vi "Draw Steering Frame Picture_Multiple Colors.vi"(5 "wheel colors":u32[](array[colorbox]), 6 "steering frame position":T1, 7 "drawing options":T2={"draw wheel states?"=FALSE, "highlight wheel index"=-1, "pixels per unit"=10.0, "draw forward velocity?"=FALSE, "velocity scale"=1.0}, 8 "error in (no error)":errorcluster, 9 "picture draw area size (pixels)":cluster{"width":u32, "height":u32}={"width"=500, "height"=500}, 10 "picture in":picture, 11 "steering frame in":refnum<class "NI_Robotics_Steering Frame.lvclass">) -> (0 "error out":errorcluster, 2 "picture out":picture, 3 "steering frame out":refnum<class "NI_Robotics_Steering Frame.lvclass">)   [LabVIEW 2017, in "NI_Robotics_Steering Picture.lvlib"]
doc: "Creates an image you can wire to a 2D picture control to visualize a steering frame on the front panel. The picture can display data about the directions and velocities at which wheels move."
uses:
  <vilib>/robotics/Utilities/Visualization/Steering Visualization/Steering Picture/NI_Robotics_Steering Picture.lvlib
  <vilib>/robotics/Steering/Steering Frame/NI_Robotics_Steering Frame.lvclass
  <vilib>/robotics/Utilities/Visualization/Steering Visualization/Steering Picture/Draw Steering Frame Options.ctl
  <vilib>/robotics/Utilities/Visualization/Steering Visualization/Steering Picture/Picture Info.ctl
  <vilib>/Utility/miscctls.llb/LVBoundsTypeDef.ctl
  <vilib>/robotics/Steering/Steering Frame/NI_Robotics_Steering Frame.lvclass/NI_Robotics_Steering Frame.ctl
  <vilib>/Analysis/coordinate.llb/2D Cartesian Coordinate Rotation (Array).vi
  <vilib>/Analysis/coordinate.llb/Angle Rotation with Same Angle (array).vi
  <vilib>/robotics/Utilities/Visualization/Steering Visualization/Steering Picture/Draw Arrow.vi
  <vilib>/robotics/Utilities/Visualization/Steering Visualization/Steering Picture/Draw Wheel Axle.vi
  <vilib>/robotics/Utilities/Visualization/Steering Visualization/Steering Picture/Draw Wheel Outline.vi
  <vilib>/robotics/Utilities/Visualization/Steering Visualization/Steering Picture/Draw Fixed Wheel Forward Velocity.vi
  <vilib>/robotics/Utilities/Visualization/Steering Visualization/Steering Picture/Draw Wedge.vi
  <vilib>/robotics/Utilities/Visualization/Steering Visualization/Steering Picture/Draw Steering Wheel Forward Velocity.vi
  <vilib>/Analysis/coordinate.llb/Angle Rotation (scalar).vi
  <vilib>/Analysis/coordinate.llb/2D Cartesian Coordinate Rotation (Scalar).vi
  <vilib>/robotics/Utilities/Visualization/Steering Visualization/Steering Picture/Global Position to Pixel.vi
  <vilib>/robotics/Utilities/Visualization/Steering Visualization/Steering Picture/Draw Caster Wheel Forward Velocity.vi
  <vilib>/robotics/Utilities/Visualization/Steering Visualization/Steering Picture/Draw Lines.vi
  <vilib>/Analysis/coordinate.llb/Wrap Angle (array).vi
  <vilib>/Analysis/coordinate.llb/Wrap Angle.vi
  <vilib>/Analysis/coordinate.llb/Wrap Angle (scalar).vi
  <vilib>/picture/picture.llb/Draw Line.vi
  <vilib>/picture/picture.llb/Move Pen.vi
  <vilib>/picture/picture.llb/Draw Point.vi
  <vilib>/picture/picture.llb/Draw Multiple Lines.vi
  <vilib>/robotics/Steering/Wheel/Get Wheel Information.vi
  <vilib>/robotics/Steering/Wheel/Get Omnidirectional Wheel Information.vi
  <vilib>/robotics/Steering/Wheel/Get Mecanum Wheel Information.vi
  <vilib>/robotics/Steering/Wheel/Get Caster Wheel Information.vi
  <vilib>/picture/pictutil.llb/Draw Circle by Radius.vi
  <vilib>/Utility/AngleManip/Radians to Degrees.vi
  <vilib>/Utility/AngleManip/Radians to Degrees (Scalar DBL).vi
  <vilib>/robotics/Steering/Wheel/Get Steering Wheel Information.vi
  <vilib>/robotics/Steering/Wheel/Get Fixed Wheel Information.vi
  <vilib>/robotics/Steering/Wheel/NI_Robotics_Wheel.lvclass
  <vilib>/Analysis/NI_AALPro.lvlib
  <vilib>/Analysis/NI_AAL_Angle.lvlib
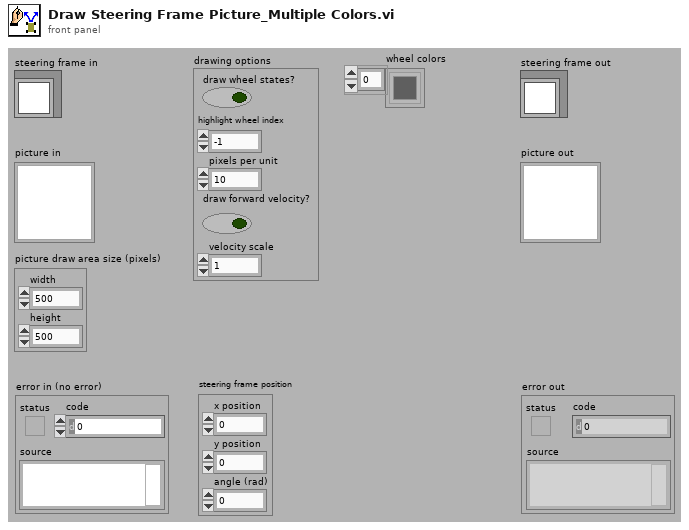
[diagram p1: front panel]
types:
  T1 = cluster{"x position":dbl, "y position":dbl, "angle (rad)":dbl}
  T2 = typedef "NI_Robotics_Steering Picture.lvlib/Draw Steering Frame Options.ctl" = cluster{"draw wheel states?":bool, "highlight wheel index":i32, "pixels per unit":dbl, "draw forward velocity?":bool, "velocity scale":dbl}
  T3 = typedef "NI_Robotics_Steering Picture.lvlib/Picture Info.ctl" = cluster{"picture size":T4, "pixels per unit":dbl}
  T4 = typedef "LVBoundsTypeDef.ctl" = cluster{"Width":u32, "Height":u32}
  T5 = typedef "NI_Robotics_Wheel.lvclass/Wheel State.ctl" = cluster{"wheel name":string, "forward angular velocity":dbl, "caster angular velocity":dbl, "caster wheel angle (rad)":dbl, "steering angle (rad)":dbl}
  T6 = typedef "NI_Robotics_Steering Picture.lvlib/Draw Wheel Options.ctl" = cluster{"global wheel position":cluster{"x":dbl, "y":dbl}, "wheel frame angle (rad)":dbl, "color (black)":u32, "draw wheel state":bool, "draw forward velocity":bool, "velocity scale":dbl, "velocity color (red)":u32}
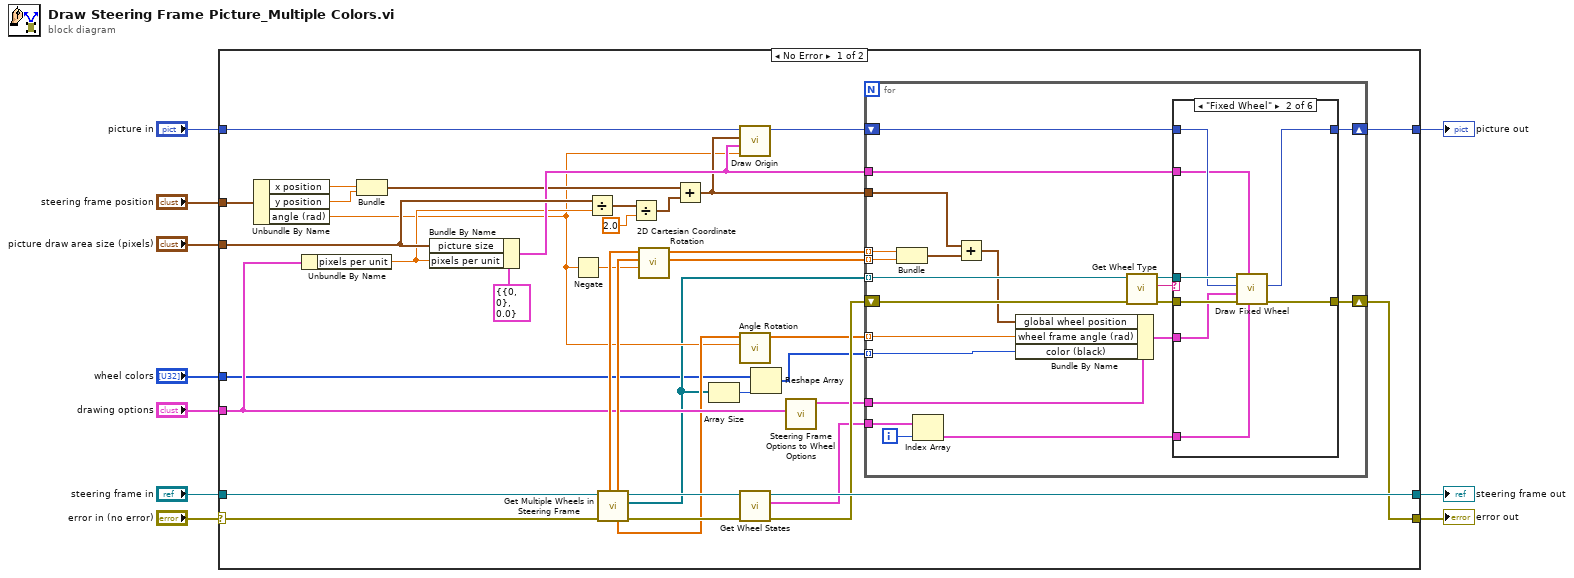
[diagram p0: block diagram]
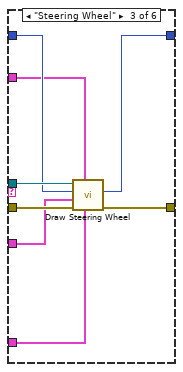
[diagram p3: hidden frame]
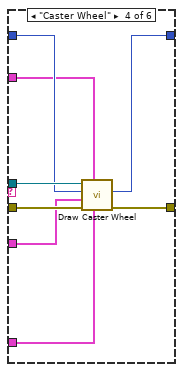
[diagram p4: hidden frame]
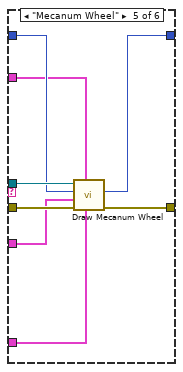
[diagram p5: hidden frame]
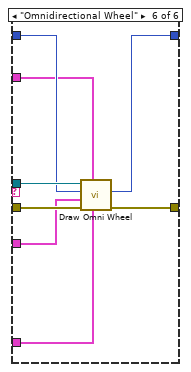
[diagram p6: hidden frame]
diagram:
  n1 = case shown="No Error" "error in (no error)" {
    selector: "error in (no error)" -> [w43 w113]
    tunnel: [w34 w113] -> w9
    tunnel: "steering frame in" -> [w45 w112]
    tunnel: [w38 w112] -> w7
    tunnel: "picture in" -> [w47 w111]
    tunnel: [w35 w111] -> w5
    tunnel: "drawing options" -> [w20 _]
    tunnel: "picture draw area size (pixels)" -> [w39 _]
    tunnel: "steering frame position" -> [w24 _]
    tunnel: "wheel colors" -> [w13 _]
    frame No Error {
      n2 = Unbundle By Name(w24) -> ("x position"=w23:dbl, "y position"=w22:dbl, "angle (rad)"=w16:dbl)
      n3 = Unbundle By Name(w20) -> ("pixels per unit"=w18:dbl)
      n4 = Bundle("x position"=w23, "y position"=w22) -> (w21:cluster{"x position":dbl, "y position":dbl})  [unwired: 1 in]
      n5 = Bundle By Name(cluster=T3 {"picture size"={"Width"=0, "Height"=0}, "pixels per unit"=0.0} ("picture info"), "picture size"=w39, "pixels per unit"=w18) -> (w32:T3)
      n6 = Negate(x=w16) -> (-x=w25:dbl)
      n7 = Divide(x=w39, y=w18) -> (x/y=w40:cluster{"width":dbl, "height":dbl})
      n8 = call <vilib>:"Get Multiple Wheels in Steering Frame.vi"("error in (no error)"=w43, "steering frame in"=w45) -> ("error out"=w42:errorcluster, "wheels"=w14:refnum<class "NI_Robotics_Wheel.lvclass">[], "steering frame out"=w44:refnum<class "NI_Robotics_Steering Frame.lvclass">, "frame angles (rad)"=w17:dbl[], "y positions"=w27:dbl[], "x positions"=w29:dbl[])  [unwired: 3 in, 1 out]
      n9 = Divide(x=w40, y=2.0) -> (x/y=w31:cluster{"width":dbl, "height":dbl})
      n10 = call-poly <vilib>:"2D Cartesian Coordinate Rotation.vi"("theta"=w25, "Y"=w27, "X"=w29) -> ("Y Out"=w26:dbl[], "X Out"=w28:dbl[])  [unwired: 6 in, 1 out]
      n11 = Add(x=w21, y=w31) -> (x+y=w30:cluster{dbl, dbl})
      n12 = Array Size(array=w14) -> (size(s)=w12:i32)
      n13 = call <vilib>:"Draw Origin.vi"("frame angle (rad)"=w16, "picture info"=w32, "frame offset position"=w30, "picture in"=w47) -> ("picture out"=w33:picture)  [unwired: 7 in]
      n14 = call-poly <vilib>:"Angle Rotation.vi"("counterclockwise rotation"=w16, "Angle"=w17) -> ("Rotated Angle"=w15:dbl[])  [unwired: 8 in, 1 out]
      n15 = call <vilib>:"Get Wheel States.vi"("error in (no error)"=w42, "steering frame in"=w44) -> ("error out"=w37:errorcluster, "wheel states"=w36:T5[], "steering frame out"=w38:refnum<class "NI_Robotics_Steering Frame.lvclass">)  [unwired: 7 in]
      n16 = Reshape Array(w13, w12) -> (w11:u32[])
      n17 = call <vilib>:"Steering Frame Options to Wheel Options.vi"("draw steering frame options"=w20) -> ("draw wheel options out"=w19:T6)  [unwired: 10 in]
      n18 = for {
        tunnel: w14 -> [w68] mode=indexing
        shift-right: [w56] -> w34
        shift-left: w37 -> [w67]
        tunnel: w26 -> [w60] mode=indexing
        tunnel: w28 -> [w61] mode=indexing
        shift-right: [w62] -> w35
        shift-left: w33 -> [w63]
        tunnel: w15 -> [w50] mode=indexing
        tunnel: w30 -> [w59]
        tunnel: w32 -> [w57]
        tunnel: w36 -> [w55]
        tunnel: w19 -> [w49]
        tunnel: w11 -> [w48] mode=indexing
        i -> [w54]
        n19 = Bundle("Numeric"=w61, "Numeric"=w60) -> (w58:cluster{"Numeric":dbl, "Numeric":dbl})  [unwired: 1 in]
        n20 = Index Array(array=w55, index=w54) -> (element=w53:T5)
        n21 = Add(x=w59, y=w58) -> (x+y=w51:cluster{dbl, dbl})
        n22 = Bundle By Name(cluster=w49, "global wheel position"=w51, "wheel frame angle (rad)"=w50, "color (black)"=w48) -> (w52:T6)
        n23 = call-dynamic "Get Wheel Type.vi"("error in (no error)"=w67, "wheel in"=w68) -> ("error out"=w65:errorcluster, "wheel type"=w66:string, "wheel out"=w64:refnum<class "NI_Robotics_Wheel.lvclass">)  [unwired: 7 in]
        n24 = case shown="\"Fixed Wheel\"" w66 {
          tunnel: w65 -> [w69 w78 w86 w94 w102 w110]
          tunnel: w64 -> [_ w76 w84 w92 w100 w108]
          tunnel: w63 -> [w70 w75 w83 w91 w99 w107]
          tunnel: [w70 w74 w82 w90 w98 w106] -> w62
          tunnel: [w69 w77 w85 w93 w101 w109] -> w56
          tunnel: w57 -> [_ w73 w81 w89 w97 w105]
          tunnel: w53 -> [_ w72 w79 w88 w95 w103]
          tunnel: w52 -> [_ w71 w80 w87 w96 w104]
          frame "Wheel", Default {
          }
          frame "Fixed Wheel" {
            n25 = call <vilib>:"Draw Fixed Wheel.vi"("wheel state"=w72, "picture info"=w73, "error in (no error)"=w78, "draw wheel options"=w71, "picture in"=w75, "wheel in"=w76) -> ("error out"=w77:errorcluster, "picture out"=w74:picture)  [unwired: 3 in, 1 out]
          }
          frame "Steering Wheel" {
            n26 = call <vilib>:"Draw Steering Wheel.vi"("wheel state"=w79, "picture info"=w81, "error in (no error)"=w86, "draw wheel options"=w80, "picture in"=w83, "wheel in"=w84) -> ("error out"=w85:errorcluster, "picture out"=w82:picture)  [unwired: 3 in, 1 out]
          }
          frame "Caster Wheel" {
            n27 = call <vilib>:"Draw Caster Wheel.vi"("wheel state"=w88, "picture info"=w89, "error in (no error)"=w94, "draw wheel options"=w87, "picture in"=w91, "wheel in"=w92) -> ("error out"=w93:errorcluster, "picture out"=w90:picture)  [unwired: 3 in, 1 out]
          }
          frame "Mecanum Wheel" {
            n28 = call <vilib>:"Draw Mecanum Wheel.vi"("wheel state"=w95, "picture info"=w97, "error in (no error)"=w102, "draw wheel options"=w96, "picture in"=w99, "wheel in"=w100) -> ("error out"=w101:errorcluster, "picture out"=w98:picture)  [unwired: 3 in, 1 out]
          }
          frame "Omnidirectional Wheel" {
            n29 = call <vilib>:"Draw Omni Wheel.vi"("wheel state"=w103, "picture info"=w105, "error in (no error)"=w110, "draw wheel options"=w104, "picture in"=w107, "wheel in"=w108) -> ("error out"=w109:errorcluster, "picture out"=w106:picture)  [unwired: 3 in, 1 out]
          }
        }
      }
    }
    frame Error {
    }
  }
  "steering frame out" <- w7
  "error out" <- w9
  "picture out" <- w5
